vi "Wait On Notification.vi"(8 "error in (no error)":errorcluster, 9 "timeout in ms (-1)":i32, 10 "ignore previous (F)":bool, 11 "observer in":T1) -> (0 "error out":errorcluster, 1 "timed out?":bool, 2 "notification":cluster{"value":variant, "name":string}, 3 "observer out":T1)   [LabVIEW 2014, in "Observable Actor.lvlib" / "Observable Actor.lvclass"]
uses:
  Observable Actor.lvclass
  Observer.ctl
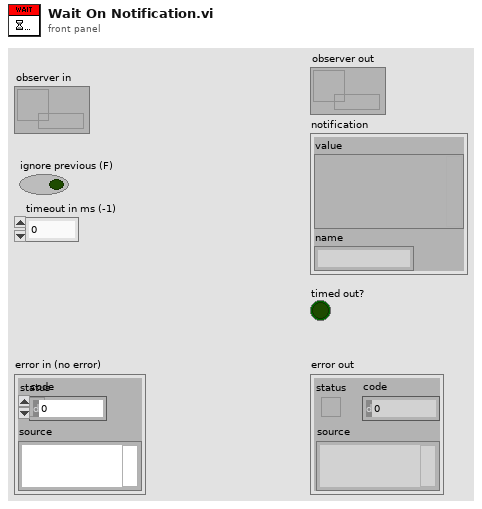
[diagram p1: front panel]
types:
  T1 = typedef "Observable Actor.lvlib/Observable Actor.lvclass/Observer.ctl" = refnum<queue>
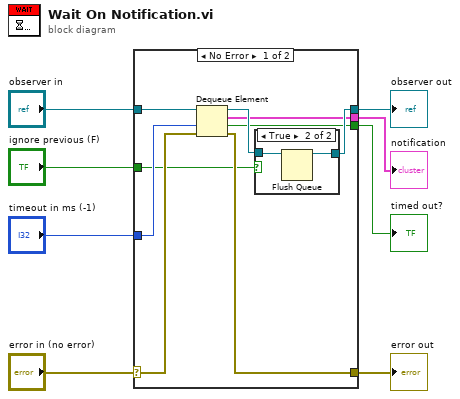
[diagram p0: block diagram]
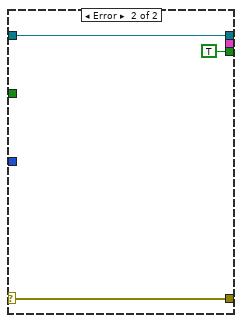
[diagram p3: hidden frame]
diagram:
  n1 = case shown="No Error" "error in (no error)" {
    selector: "error in (no error)" -> [w14 w23]
    tunnel: [w16 w23] -> w7
    tunnel: "observer in" -> [w17 w22]
    tunnel: "ignore previous (F)" -> [w11 _]
    tunnel: "timeout in ms (-1)" -> [w15 _]
    tunnel: [w12 w22] -> w3
    tunnel: [w10 _] -> w2
    tunnel: [w9 TRUE ("timed out?")] -> w1
    frame No Error {
      n2 = Dequeue Element(queue=w17, timeout in ms (-1)=w15, error in (no error)=w14) -> (queue out=w13:T1, element=w10:cluster{"value":variant, "name":string}, timed out?=w9:bool, error out=w16:errorcluster)
      n3 = case shown="True" w11 {
        tunnel: w13 -> [w18 w20]
        tunnel: [w18 w19] -> w12
        frame False {
        }
        frame True {
          n4 = Flush Queue(queue=w20) -> (queue out=w19:T1)  [unwired: 1 in, 2 out]
        }
      }
    }
    frame Error {
    }
  }
  "error out" <- w7
  "observer out" <- w3
  "notification" <- w2
  "timed out?" <- w1
